vi "DAQ_Analog_Initialize.vi"(8 "error in (no error)":errorcluster, 11 "task/channels in":refnum<k21>="Photodetectors") -> (0 "error out":errorcluster, 3 "task out":refnum<k21>)   [LabVIEW 2018]
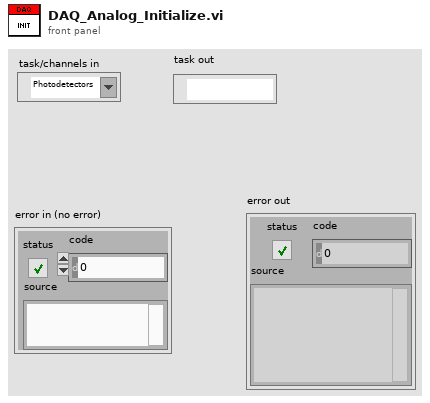
[diagram p1: front panel]
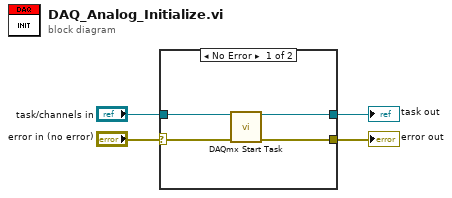
[diagram p0: block diagram]
diagram:
  n1 = case shown="No Error" "error in (no error)" {
    selector: "error in (no error)" -> [w8 w9]
    tunnel: [w7 w9] -> w3
    tunnel: [w6 w10] -> w2
    tunnel: "task/channels in" -> [w5 w10]
    frame No Error {
      n2 = call "DAQmx Start Task.vi"("task/channels in"=w5, "error in"=w8) -> ("task out"=w6:refnum<k21>, "error out"=w7:errorcluster)  [unwired: 12 in]
    }
    frame Error {
    }
  }
  "error out" <- w3
  "task out" <- w2
